vi "Day01-06.vi"() -> ()   [LabVIEW 2021]
panel:
  out "구구단":i32[][](array[numeric])
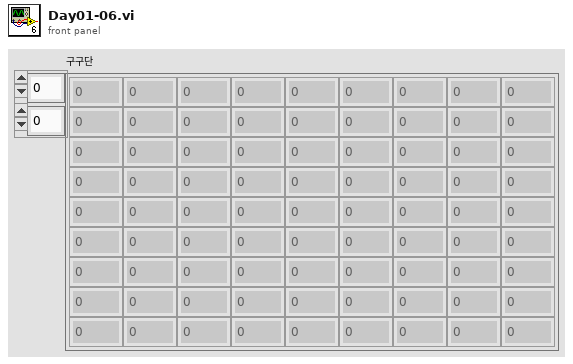
[diagram p1: front panel]
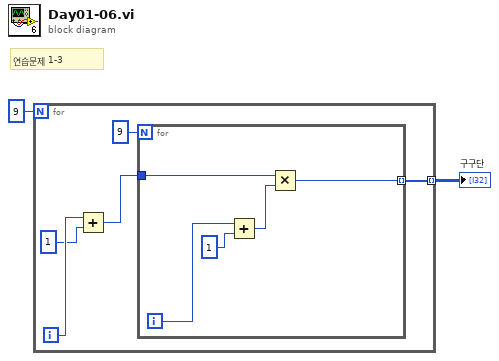
[diagram p0: block diagram]
diagram:
  # "연습문제 1-3"
  n1 = for {
    N: 9 -> [_]
    tunnel: [w3] -> w1 mode=indexing
    i -> [w6]
    n2 = Add(x=w6, y=1) -> (x+y=w4:i32)
    n3 = for {
      N: 9 -> [_]
      tunnel: w4 -> [w10]
      tunnel: [w8] -> w3 mode=indexing
      i -> [w12]
      n4 = Add(x=w12, y=1) -> (x+y=w9:i32)
      n5 = Multiply(x=w10, y=w9) -> (x*y=w8:i32)
    }
  }
  "구구단" <- w1
